vi "Switch Initialization.vi"(8 "error in (no error)":errorcluster, 11 "Configurations":T1={"Common RFout"="PXI1Slot9", "Port1 Incident"="COM", "Port2 Incident"="CH1", "Port1 Reference"="CH2", "Port1 Test"="CH6", "Common RFin"="CH1", "Port2 Reference"="COM", "Port2 Test"="PXI1Slot12", "RF Out Switch"="CH5", "RF In Switch"="CH4"}) -> (0 "error out":errorcluster, 3 "SParam Switch Reference":refnum<data-value>)   [LabVIEW 2023, in "FPT_SParam_Switching.lvclass"]
uses:
  FPT_SParam_Switching.lvclass
  FPT_SParam_Switching.lvclass/FPT_SParam_Switching.ctl
  Switch Configuration.ctl
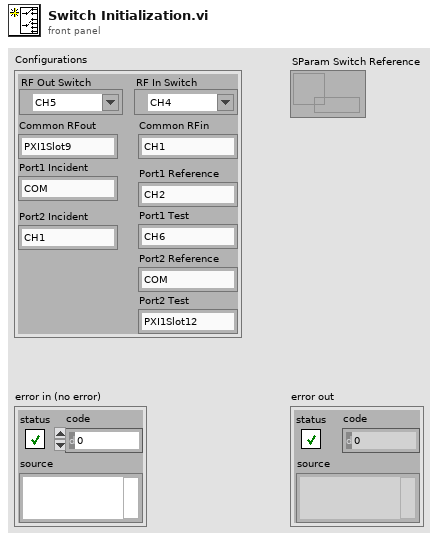
[diagram p1: front panel]
types:
  T1 = typedef "FPT_SParam_Switching.lvclass/Switch Configuration.ctl" = cluster{"Common RFout":string, "Port1 Incident":string, "Port2 Incident":string, "Port1 Reference":string, "Port1 Test":string, "Common RFin":string, "Port2 Reference":string, "Port2 Test":string, "RF Out Switch":refnum<k15>, "RF In Switch":refnum<k15>}
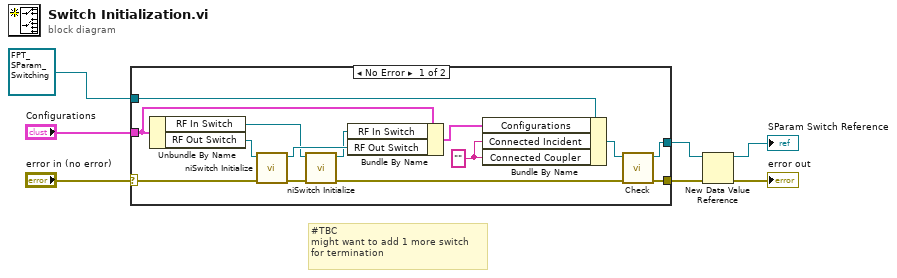
[diagram p0: block diagram]
diagram:
  # "#TBC\nmight want to add 1 more switch\nfor termination"
  n1 = case shown="No Error" "error in (no error)" {
    selector: "error in (no error)" -> [w20 w23]
    tunnel: [w10 w23] -> w4
    tunnel: refnum<class "FPT_SParam_Switching.lvclass"> refnum ("FPT_SParam_Switching.lvclass") -> [w14 w22]
    tunnel: "Configurations" -> [w15 _]
    tunnel: [w8 w22] -> w5
    frame No Error {
      w12 = "" ("Connected Incident")
      n2 = Unbundle By Name(w15) -> ("RF In Switch"=w16:refnum<k15>, "RF Out Switch"=w17:refnum<k15>)
      n3 = call <instrlib>:"niSwitch Initialize.vi"("error in (no error)"=w20, "resource name"=w17) -> ("error out"=w19:errorcluster, "instrument handle out"=w21:refnum<k15>)  [unwired: 8 in]
      n4 = call <instrlib>:"niSwitch Initialize.vi"("error in (no error)"=w19, "resource name"=w16) -> ("error out"=w11:errorcluster, "instrument handle out"=w18:refnum<k15>)  [unwired: 8 in]
      n5 = Bundle By Name(cluster=w15, "RF In Switch"=w18, "RF Out Switch"=w21) -> (w13:T1)
      n6 = Bundle By Name(cluster=w14, "Configurations"=w13, "Connected Incident"=w12, "Connected Coupler"=w12) -> (w9:refnum<class "FPT_SParam_Switching.lvclass">)
      n7 = call "Check.vi"("error in (no error)"=w11, "FPT_SParam_Switching in"=w9) -> ("error out"=w10:errorcluster, "FPT_SParam_Switching out"=w8:refnum<class "FPT_SParam_Switching.lvclass">)  [unwired: 8 in]
    }
    frame Error {
    }
  }
  n8 = New Data Value Reference(data value=w5, error in=w4) -> (data value reference=→"SParam Switch Reference":refnum<data-value>, error out=→"error out":errorcluster)
